vi "Init.vi"(8 "Error In":errorcluster, 11 "Mark All Errors As Read Button Reference":refnum<vi>) -> (0 "Error Out":errorcluster)   [LabVIEW 2023, in "Error Manager.lvlib" / "Mark All Errors As Read Button.lvclass"]
doc: "Blank VI with error handling."
uses:
  Mark All Errors As Read Button.lvclass
  Mark All Errors As Read Button.lvclass/Mark All Errors As Read Button.ctl
panel:
  # "Input\nInputs to the VI"
  # "Development\nControls or indicators that are useful for development or testing, but which are not outputs of the VI."
  # "Output\nOutputs of the VI"
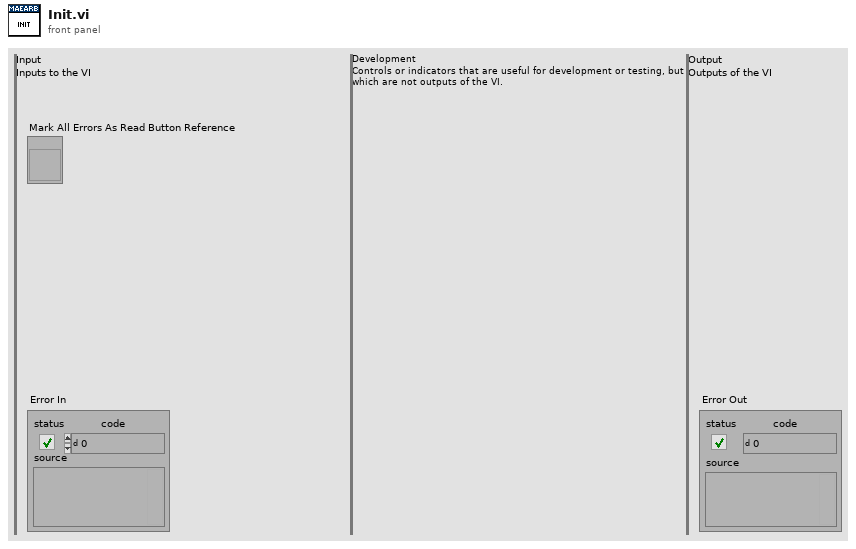
[diagram p1: front panel]
types:
  T1 = enum8{"Enabled", "Disabled", "Disabled and Grayed Out"}
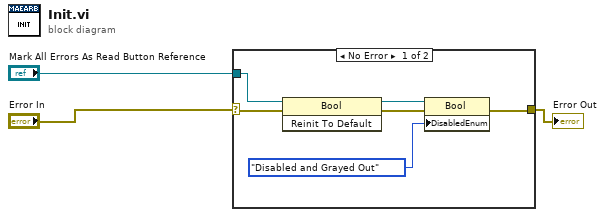
[diagram p0: block diagram]
diagram:
  n1 = case shown="No Error" "Error In" {
    selector: "Error In" -> [w9 w10]
    tunnel: [w8 w10] -> w2
    tunnel: "Mark All Errors As Read Button Reference" -> [w5 _]
    frame No Error {
      n2 = invoke class="Bool" method="Reinit To Default"(reference=w5, error in=w9) -> (reference out=w4:refnum<vi>, error out=w6:errorcluster)  [unwired: 1 in, 1 out]
      n3 = property class="Bool"(reference=w4, error in=w6, "DisabledEnum"=T1."Disabled and Grayed Out" ("Disabled")) -> (error out=w8:errorcluster)  [unwired: 1 out]
    }
    frame Error {
    }
  }
  "Error Out" <- w2
